vi "ATF-Pump-Glitch_Remove1_A.vi"(11 "Input":dbl format="%#_13g") -> (3 "Output":dbl)   [LabVIEW 2022 SP3]
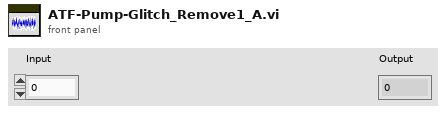
[diagram p1: front panel]
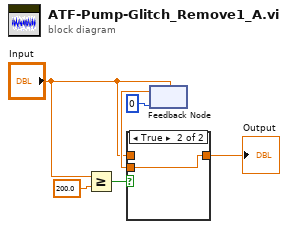
[diagram p0: block diagram]
diagram:
  n1 = Greater Or Equal?(x="Input", y=200.0) -> (x >= y?=w5:bool)
  n2 = feedback #1(0 ("Input")) -> (w4:dbl)
  n3 = case shown="True" w5 {
    tunnel: "Input" -> [w7 _]
    tunnel: [w7 w8] -> w2
    tunnel: w4 -> [_ w8]
    frame False {
    }
    frame True {
    }
  }
  "Output" <- w2
  n4 = feedback-in #1("Input") -> ()
